vi "pu_to_unp.vi"(1 "x":i16) -> (0 "y":T1)   [LabVIEW 2018, in "posit.lvlib"]
uses:
  posit.lvlib
  unpacked.ctl
  specialnumber.ctl
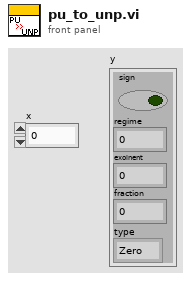
[diagram p1: front panel]
types:
  T1 = typedef "posit.lvlib/unpacked.ctl" = cluster{"sign":bool, "regime":i16, "exoinent":i16, "fraction":i16, "type":T2}
  T2 = typedef "posit.lvlib/specialnumber.ctl" = enum16{"Zero", "Regular", "NaN", "Infinity"}
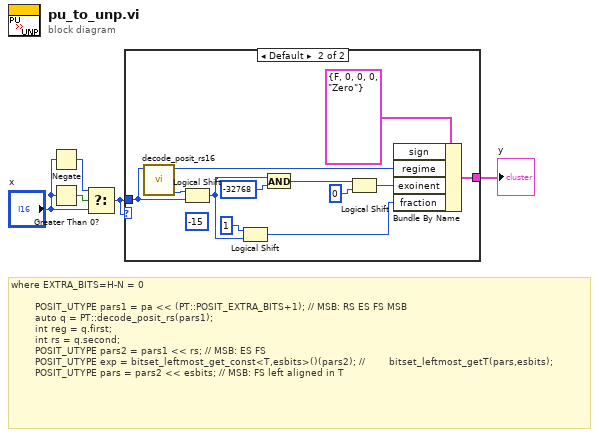
[diagram p0: block diagram]
diagram:
  # "where EXTRA_BITS=H-N = 0\n\n        POSIT_UTYPE pars1 = pa << (PT::POSIT_EXTRA_BITS+1); // MSB: RS ES FS MSB\n        auto q = PT::decode_posit_rs(pars1);\n        int reg = q.first;\n        int rs = q.second;\n        POSIT_UTYPE pars2 = pars1 << rs; // MSB: ES FS\n        POSIT_UTYPE exp = bitset_leftmost_get_const<T,esbits>()(pars2); //        bitset_leftmost_getT(pars,esbits);\n        POSIT_UTYPE pars = pars2 << esbits; // MSB: FS left aligned in T"
  n1 = Negate(x="x") -> (-x=w4:i16)
  n2 = Greater Than 0?(x="x") -> (x > 0?=w5:bool)
  n3 = Select(t=w4, s=w5, f="x") -> (s? t:f=w2:i16)
  n4 = case shown="Default" w2 {
    tunnel: w2 -> [_ w14]
    tunnel: [_ w7] -> w1
    frame 0 {
    }
    frame Default {
      (unwired) i16 -15 ("x << y")
      n5 = call "decode_posit_rs16.vi"("pars"=w14) -> ("rs"=w15:i16, "reg"=w16:i16)  [unwired: 9 in]
      n6 = Logical Shift(y=w15, x=w14) -> (x << y=w10:i16)
      n7 = Logical Shift(y=i16 1, x=w10) -> (x << y=w12:i16)
      n8 = And(x=w10, y=i16 -32768) -> (x .and. y?=w9:i16)
      n9 = Logical Shift(y=w9, x=i16 0) -> (x << y=w8:i16)
      n10 = Bundle By Name(cluster=T1 {"sign"=FALSE, "regime"=0, "exoinent"=0, "fraction"=0, "type"=enum."Zero"} ("y 2"), "regime"=w16, "exoinent"=w8, "fraction"=w12) -> (w7:T1)  [unwired: 1 in]
    }
  }
  "y" <- w1
